vi "Log gRPC Error.vi"(8 "error IO":errorcluster, 11 "gRPC ID in":T1) -> (0 "error out":errorcluster, 3 "gRPCid out":T1)   [LabVIEW 2021, in "NI DAQmx_wrapper.lvlib"]
uses:
  NI DAQmx_wrapper.lvlib
  <vilib>/gRPC/LabVIEW gRPC Library/Shared/grpcId.ctl
  <vilib>/gRPC/LabVIEW gRPC Library/Server API/typeDefs/gRPC Status Code.ctl
  <vilib>/Utility/error.llb/DialogType.ctl
  <vilib>/gRPC/LabVIEW gRPC Library/grpc-lvsupport-release.lvlib
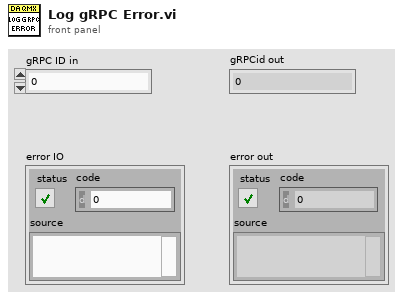
[diagram p1: front panel]
types:
  T1 = typedef "grpc-lvsupport-release.lvlib/grpcId.ctl" = u64
  T2 = typedef "grpc-lvsupport-release.lvlib/gRPC Status Code.ctl" = enum16{"OK", "CANCELLED", "UNKNOWN", "INVALID_ARGUMENT", "DEADLINE_EXCEEDED", "NOT_FOUND", "ALREADY_EXISTS", "PERMISSION_DENIED", "RESOURCE_EXHAUSTED", "FAILED_PRECONDITION", "ABORTED", "OUT_OF_RANGE", "UNIMPLEMENTED", "INTERNAL", "UNAVAILABLE", "DATA_LOSS", "UNAUTHENTICATED"}
  T3 = typedef "DialogType.ctl" = u16
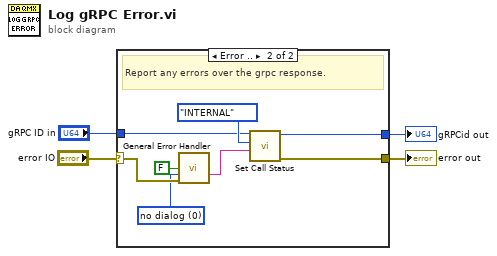
[diagram p0: block diagram]
diagram:
  n1 = case shown="Error .." "error IO" {
    selector: "error IO" -> [w6 w11]
    tunnel: [w6 w13] -> w2
    tunnel: "gRPC ID in" -> [w5 w12]
    tunnel: [w5 w7] -> w1
    frame No Error {
      # "no error: pass through"
    }
    frame Error {
      w9 = T3 0 items=["no dialog", "OK message", "continue or stop message", "OK message + warnings", "continue/stop + warnings"] ("type of dialog (OK msg:1)")
      # "Report any errors over the grpc response."
      n2 = call <vilib>:"General Error Handler.vi"("search ni.com link visible?(T)"=FALSE, "type of dialog (OK msg:1)"=w9, "error in (no error)"=w11) -> ("message"=w10:string)  [unwired: 8 in, 4 out]
      n3 = call <vilib>:"Set Call Status.vi"("Details"=w10, "Status Code"=gRPC_Status_Code."INTERNAL", "gRPCid in"=w12) -> ("error out"=w13:errorcluster, "gRPCid out"=w7:T1)  [unwired: 7 in]
    }
  }
  "error out" <- w2
  "gRPCid out" <- w1
